vi "CaritaOficial.vi"() -> ()   [LabVIEW 2018]
panel:
  out "Carita":bool[][](array[boolean])
  in  "Escoje un numero del 0 al 10":dbl
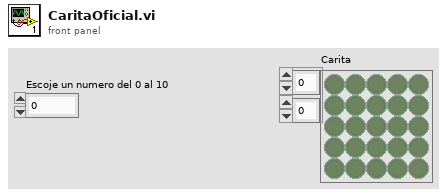
[diagram p1: front panel]
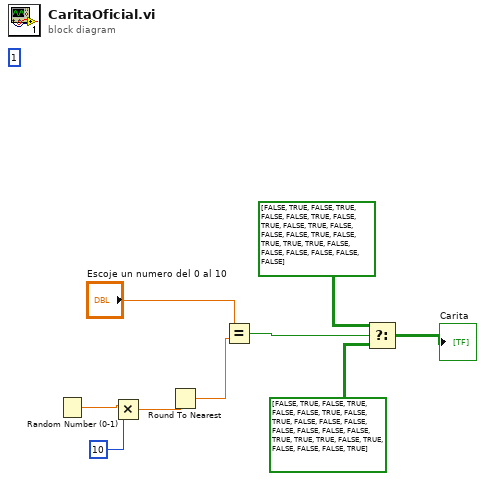
[diagram p0: block diagram]
diagram:
  (unwired) 1
  n1 = Random Number (0-1)() -> (number: 0 to 1=w6:dbl)
  n2 = Multiply(x=w6, y=10) -> (x*y=w5:dbl)
  n3 = Round To Nearest(number=w5) -> (nearest integer value=w4:dbl)
  n4 = Equal?(x="Escoje un numero del 0 al 10", y=w4) -> (x = y?=w3:bool)
  n5 = Select(t=bool[][] [[FALSE, TRUE, FALSE, TRUE, FALSE], [FALSE, TRUE, FALSE, TRUE, FALSE], [TRUE, FALSE, FALSE, FALSE, TRUE], [FALSE, TRUE, TRUE, TRUE, FALSE], [FALSE, FALSE, FALSE, FALSE, FALSE]], s=w3, f=bool[][] [[FALSE, TRUE, FALSE, TRUE, FALSE], [FALSE, TRUE, FALSE, TRUE, FALSE], [FALSE, FALSE, FALSE, FALSE, FALSE], [FALSE, TRUE, TRUE, TRUE, FALSE], [TRUE, FALSE, FALSE, FALSE, TRUE]]) -> (s? t:f=→"Carita":bool[][])
